vi "IDS_system_getAxisSignalQuality.vi"(0 "deviceHandle":i32, 2 "axisNumber":i32, 3 "error in (no error)":errorcluster) -> (7 "deviceHandle out":i32, 8 "contrast out":i32, 9 "baseline out":i32, 10 "error out":errorcluster)   [LabVIEW 2016]
panel:
  in  "baseline":i32
  in  "quality":i32
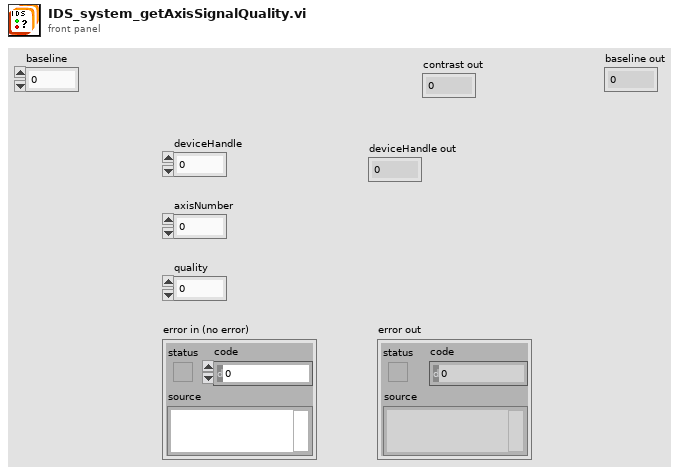
[diagram p1: front panel]
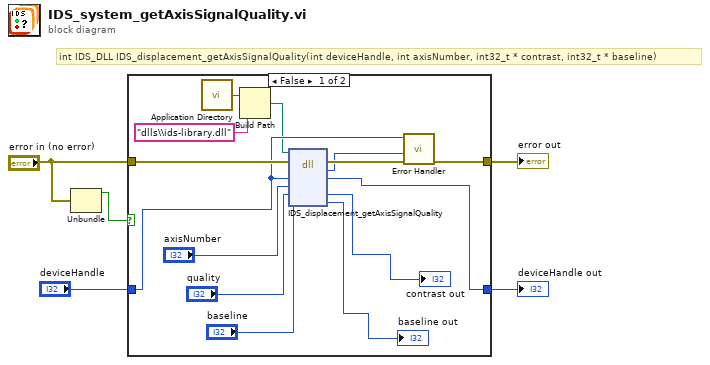
[diagram p0: block diagram]
diagram:
  # "int IDS_DLL IDS_displacement_getAxisSignalQuality(int deviceHandle, int axisNumber, int32_t * contrast, int32_t * baseline)"
  n1 = Unbundle("error in (no error)") -> ("status"=w1:bool)  [unwired: 2 out]
  n2 = case shown="False" w1 {
    tunnel: "error in (no error)" -> [w16 w21]
    tunnel: [w14 w21] -> w5
    tunnel: "deviceHandle" -> [w11 w20]
    tunnel: [w13 w20] -> w3
    frame False {
      n3 = call <vilib>:"Application Directory.vi"() -> ("Application Directory"=w8:path)
      n4 = Build Path(base path=w8, name or relative path="dlls\\ids-library.dll" ("ipAddress")) -> (appended path=w6:path)
      n5 = dll-call lib="C:/Users/matheus/Desktop/LabVIEW_Draft_V1.6.0/dlls/ids-library.dll" fn="IDS_displacement_getAxisSignalQuality"(path in=w6, error in=w16, "deviceHandle"=w11, "axisNumber"="axisNumber", "contrast"="quality", "baseline"="baseline") -> (error out=w15:errorcluster, "Rückgabetyp"=w12:i32, "deviceHandle"=w13:i32, "contrast"=→"contrast out":i32, "baseline"=→"baseline out":i32)  [unwired: 2 in, 1 out]
      n6 = call "Error Handler.vi"("error in (no error)"=w15, "error code"=w12, "deviceHandle"=w11) -> ("error out"=w14:errorcluster)  [unwired: 7 in, 1 out]
    }
    frame True {
    }
  }
  "error out" <- w5
  "deviceHandle out" <- w3
